vi "shooter_getcmds.vi"(11 "Joysticks":T5) -> (3 "Shooter":T3)   [LabVIEW 2012]
uses:
  <vilib>/Rock Robotics/WPI/Joystick/WPI_JoystickButtonState.ctl
  shooter_cmds.ctl
  <vilib>/Rock Robotics/WPI/CAN/Jaguar/SubVIs/WPI_CANJaguar_StatusSelect.ctl
  <vilib>/Rock Robotics/WPI/CAN/Jaguar/SubVIs/WPI_CANJaguar_Status.ctl
  <vilib>/Rock Robotics/WPI/CAN/Jaguar/SubVIs/WPI_CANJaguar_StatusChannelSelect.ctl
  <vilib>/ptbypt/NI_PtbyPt.lvlib
panel:
  out "Status":T1 {"Fault Counters"."CAN Status" format="%.0x"}
  in  "Status Select":T2[](array[typedef])=[enum."Output Voltage"]
  out "error out":errorcluster
  in  "Const":dbl
  in  "Coeff":dbl=1.0
  in  "Shooter 2":T3
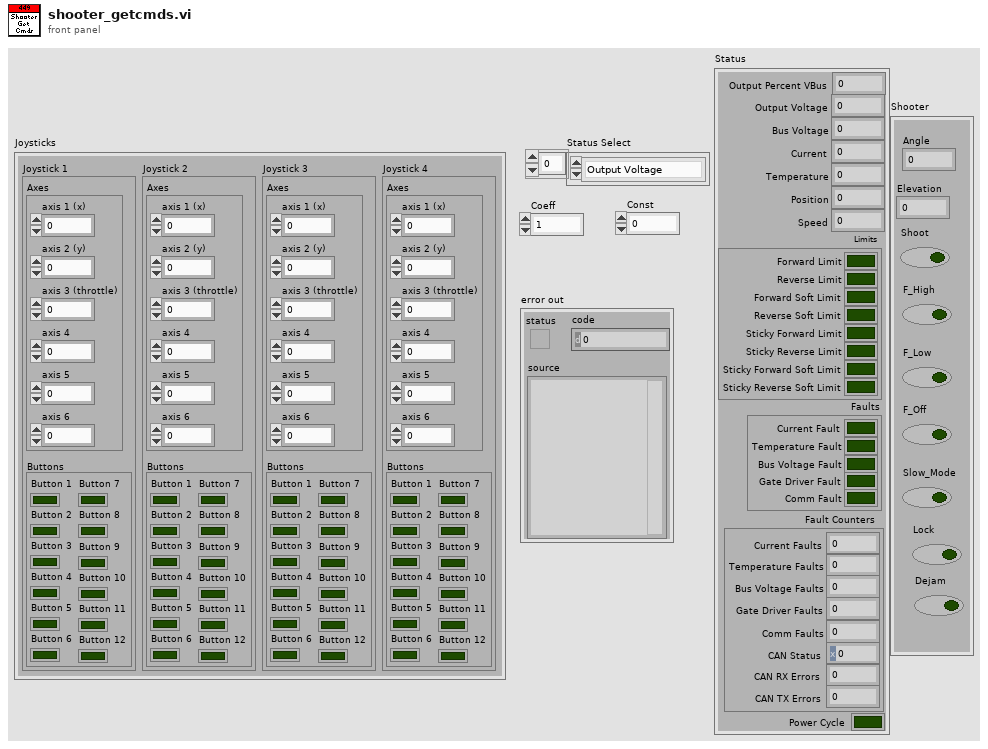
[diagram p1: front panel]
types:
  T1 = typedef "WPI_CANJaguar_Status.ctl" = cluster{"Output Percent VBus":dbl, "Output Voltage":dbl, "Bus Voltage":dbl, "Current":dbl, "Temperature":dbl, "Position":dbl, "Speed":dbl, "Limits":cluster{"Forward Limit":bool, "Reverse Limit":bool, "Forward Soft Limit":bool, "Reverse Soft Limit":bool, "Sticky Forward Limit":bool, "Sticky Reverse Limit":bool, "Sticky Forward Soft Limit":bool, "Sticky Reverse Soft Limit":bool}, "Faults":cluster{"Current Fault":bool, "Temperature Fault":bool, "Bus Voltage Fault":bool, "Gate Driver Fault":bool, "Comm Fault":bool}, "Fault Counters":cluster{"Current Faults":u8, "Temperature Faults":u8, "Bus Voltage Faults":u8, "Gate Driver Faults":u8, "Comm Faults":u8, "CAN Status":u8, "CAN RX Errors":u8, "CAN TX Errors":u8}, "Power Cycle":bool}
  T2 = typedef "WPI_CANJaguar_StatusSelect.ctl" = enum16{"Output Percent VBus", "Output Voltage", "Bus Voltage", "Current", "Temperature", "Position", "Speed", "Limit Switches", "Faults", "Fault Counters", "Power Cycle"}
  T3 = typedef "shooter_cmds.ctl" = cluster{"Elevation":dbl, "Shoot":bool, "F_High":bool, "F_Low":bool, "F_Off":bool, "Slow_Mode":bool, "Lock":bool, "Dejam":bool, "Angle":dbl}
  T4 = typedef "WPI_JoystickButtonState.ctl" = cluster{"Button 1":bool, "Button 2":bool, "Button 3":bool, "Button 4":bool, "Button 5":bool, "Button 6":bool, "Button 7":bool, "Button 8":bool, "Button 9":bool, "Button 10":bool, "Button 11":bool, "Button 12":bool}
  T5 = cluster{"Joystick 1":cluster{"Axes":cluster{"axis 1 (x)":dbl, "axis 2 (y)":dbl, "axis 3 (throttle)":dbl, "axis 4":dbl, "axis 5":dbl, "axis 6":dbl}, "Buttons":T4}, "Joystick 2":cluster{"Axes":cluster{"axis 1 (x)":dbl, "axis 2 (y)":dbl, "axis 3 (throttle)":dbl, "axis 4":dbl, "axis 5":dbl, "axis 6":dbl}, "Buttons":T4}, "Joystick 3":cluster{"Axes":cluster{"axis 1 (x)":dbl, "axis 2 (y)":dbl, "axis 3 (throttle)":dbl, "axis 4":dbl, "axis 5":dbl, "axis 6":dbl}, "Buttons":T4}, "Joystick 4":cluster{"Axes":cluster{"axis 1 (x)":dbl, "axis 2 (y)":dbl, "axis 3 (throttle)":dbl, "axis 4":dbl, "axis 5":dbl, "axis 6":dbl}, "Buttons":T4}}
  T6 = typedef "WPI_CANJaguar_StatusChannelSelect.ctl" = enum16{"Periodic Status Channel 1", "Periodic Status Channel 2", "Periodic Status Channel 3", "Periodic Status Channel 4", "On Demand Status"}
  T7 = cluster{"Axes":cluster{"axis 1 (x)":dbl, "axis 2 (y)":dbl, "axis 3 (throttle)":dbl, "axis 4":dbl, "axis 5":dbl, "axis 6":dbl}, "Buttons":T4}
  T8 = cluster{"axis 1 (x)":dbl, "axis 2 (y)":dbl, "axis 3 (throttle)":dbl, "axis 4":dbl, "axis 5":dbl, "axis 6":dbl}
  T9 = typedef "WPI_MotorControlDeviceRef.ctl" = cluster{"DeviceStatus":errorcluster, "Type":enum16{"PWM", "CAN"}, "PWM":cluster{"Digital Module":T10, "PWM Channel":T11, "DeadBand":T12}, "CAN":cluster{"Device Number":u8, "Control Mode":T13, "Semaphore":T14, "Max Vout":dbl}, "Invert":bool, "TransformRef":T15, "InvTransformRef":T15}
  T10 = typedef "FPGA_TypedefDigitalModule.ctl" = enum16{"Digital Module 1", "Digital Module 2"}
  T11 = typedef "FPGA_DIOPWMChannel.ctl" = enum8{"PWM 1", "PWM 2", "PWM 3", "PWM 4", "PWM 5", "PWM 6", "PWM 7", "PWM 8", "PWM 9", "PWM 10", "Invalid"}
  T12 = typedef "WPI_PWMDeadband.ctl" = cluster{"Name":string, "maxPositivePwm":i32, "minPositivePwm":i32, "centerPwm":i32, "maxNegativePwm":i32, "minNegativePwm":i32, "angularRange":u16}
  T13 = typedef "WPI_CANJaguar_ControlMode.ctl" = enum8{"Percent VBus", "Current", "Speed", "Position", "Voltage"}
  T14 = typedef "Semaphore RefNum" = refnum<k1>
  T15 = typedef "WPI_PWMTransform_ConPane.ctl" = refnum<vi>
  T16 = typedef "WPI_AnalogChannelDevRef.ctl" = cluster{"DevStatus":errorcluster, "Analog Module":T17, "Analog Channel":T18}
  T17 = typedef "FPGA_TypedefAnalogModule.ctl" = enum16{"Analog Module 1", "Analog Module 2"}
  T18 = typedef "FPGA_AIChannel.ctl" = enum8{"AI 1", "AI 2", "AI 3", "AI 4", "AI 5", "AI 6", "AI 7", "AI 8", "Invalid"}
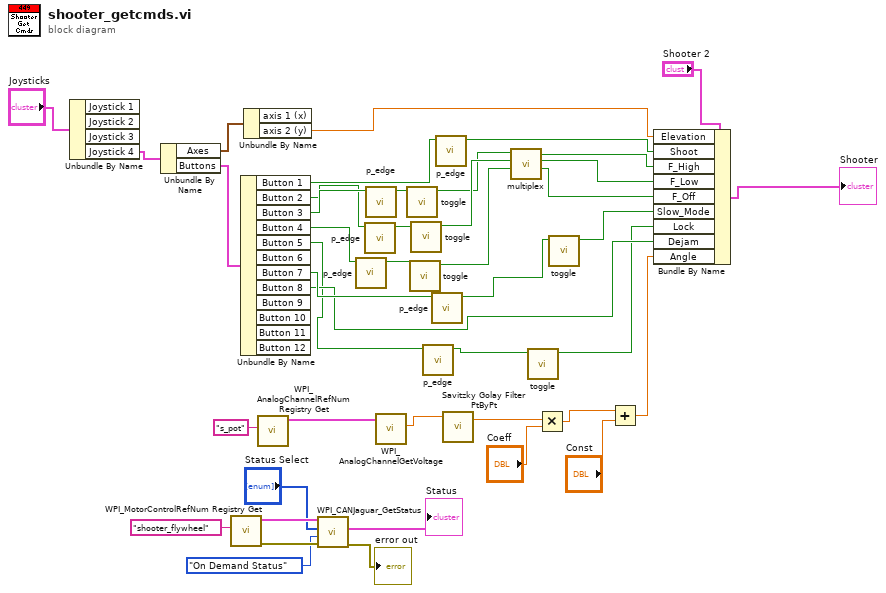
[diagram p0: block diagram]
diagram:
  n1 = Unbundle By Name("Joysticks") -> ("Joystick 4"=w42:T7)  [unwired: 3 out]
  n2 = Unbundle By Name(w42) -> ("Axes"=w41:T8, "Buttons"=w40:T4)
  n3 = call <vilib>:"WPI_MotorControlRefNum Registry Get.vi"("refnum name"="shooter_flywheel") -> ("error out"=w5:errorcluster, "MotorControlDevRef"=w7:T9)  [unwired: 9 in]
  n4 = Unbundle By Name(w40) -> ("Button 1"=w39:bool, "Button 2"=w21:bool, "Button 3"=w22:bool, "Button 4"=w31:bool, "Button 5"=w16:bool, "Button 7"=w38:bool, "Button 8"=w24:bool)  [unwired: 5 out]
  n5 = Unbundle By Name(w41) -> ("axis 2 (y)"=w23:dbl)  [unwired: 1 out]
  n6 = call <vilib>:"WPI_AnalogChannelRefNum Registry Get.vi"("refnum name"="s_pot") -> ("AIDeviceRef"=w14:T16)  [unwired: 9 in, 1 out]
  n7 = call <vilib>:"WPI_CANJaguar_GetStatus.vi"("error in (no error)"=w5, "Status Channel Select"=WPI_CANJaguar_StatusChannelSelect."On Demand Status", "Status Select"="Status Select", "CAN Jaguar Ref"=w7) -> ("error out"=→"error out":errorcluster, "Status"=→"Status":T1)  [unwired: 5 in, 1 out]
  n8 = call "p_edge.vi"("In"=w31) -> ("Out"=w35:bool)  [unwired: 10 in]
  n9 = call "p_edge.vi"("In"=w21) -> ("Out"=w36:bool)  [unwired: 10 in]
  n10 = call "p_edge.vi"("In"=w22) -> ("Out"=w37:bool)  [unwired: 10 in]
  n11 = call <vilib>:"WPI_AnalogChannelGetVoltage.vi"("AIDeviceRef"=w14) -> ("Voltage"=w13:dbl)  [unwired: 8 in, 2 out]
  n12 = call "toggle.vi"("In"=w37) -> ("Out"=w32:bool)  [unwired: 10 in]
  n13 = call "toggle.vi"("In"=w35) -> ("Out"=w34:bool)  [unwired: 10 in]
  n14 = call "toggle.vi"("In"=w36) -> ("Out"=w33:bool)  [unwired: 10 in]
  n15 = call "p_edge.vi"("In"=w16) -> ("Out"=w18:bool)  [unwired: 10 in]
  n16 = call "p_edge.vi"("In"=w38) -> ("Out"=w20:bool)  [unwired: 10 in]
  n17 = call "p_edge.vi"("In"=w39) -> ("Out"=w26:bool)  [unwired: 10 in]
  n18 = call <vilib>:"Savitzky Golay Filter PtByPt.vi"("x"=w13) -> ("Filtered x"=w12:dbl)  [unwired: 3 in, 1 out]
  n19 = call "multiplex.vi"("in 3"=w34, "in 2"=w33, "in 1"=w32) -> ("out 3"=w29:bool, "out 2"=w28:bool, "out 1"=w27:bool)  [unwired: 6 in]
  n20 = call "toggle.vi"("In"=w18) -> ("Out"=w17:bool)  [unwired: 10 in]
  n21 = Multiply(x=w12, y="Coeff") -> (x*y=w10:dbl)
  n22 = call "toggle.vi"("In"=w20) -> ("Out"=w19:bool)  [unwired: 10 in]
  n23 = Add(x=w10, y="Const") -> (x+y=w8:dbl)
  n24 = Bundle By Name(cluster="Shooter 2", "Elevation"=w23, "Shoot"=w26, "F_High"=w27, "F_Low"=w28, "F_Off"=w29, "Slow_Mode"=w19, "Lock"=w17, "Dejam"=w24, "Angle"=w8) -> (→"Shooter":T3)
